vi "Read JSON from File.vi"(8 "error in (no error)":errorcluster, 11 "File Path":path) -> (0 "error out":errorcluster, 3 "<JSON>Config":string)   [LabVIEW 2023, in "HAL GOOP4.lvlib" / "Measure and Stimulus Subsystems.lvclass"]
uses:
  Measure and Stimulus Subsystems.lvclass
  <vilib>/Utility/error.llb/Error Cluster From Error Code.vi
  <vilib>/ErrorRing/Error Ring.xnode
  Measure and Stimulus Subsystems.lvclass/Measure and Stimulus Subsystems.ctl
  <vilib>/JDP Science/JSONtext/Config Files/Config File.lvclass
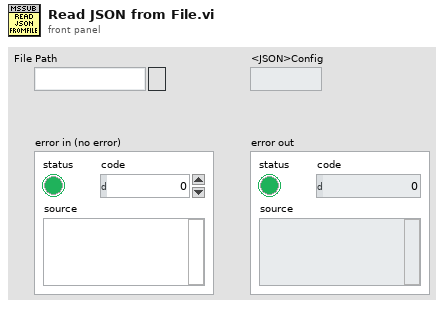
[diagram p1: front panel]
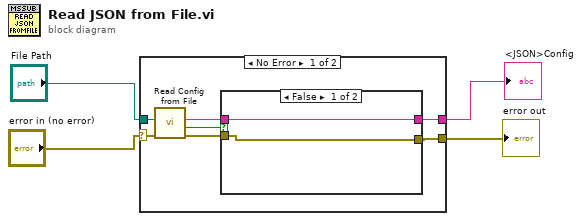
[diagram p0: block diagram]
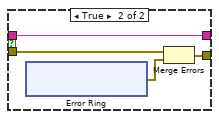
[diagram p2: hidden frame]
diagram:
  n1 = case shown="No Error" "error in (no error)" {
    selector: "error in (no error)" -> [w5 w23]
    tunnel: [w11 w23] -> w4
    tunnel: [w10 _] -> w3
    tunnel: "File Path" -> [w6 _]
    frame No Error {
      n2 = call <vilib>:"Read Config from File.vi"("error in (no error)"=w5, "config file path"=w6) -> ("error out"=w8:errorcluster, "Template Used (file missing or corrupted)"=w7:bool, "<JSON>Config"=w9:string)  [unwired: 6 in, 1 out]
      n3 = case shown="False" w7 {
        tunnel: w8 -> [w13 w17]
        tunnel: [w13 w15] -> w11
        tunnel: w9 -> [w12 w14]
        tunnel: [w12 w14] -> w10
        frame False {
        }
        frame True {
          n4 = xnode "Error Ring"() -> ("error out"=w16:errorcluster)
          n5 = Merge Errors(w17, w16) -> (w15:errorcluster)
        }
      }
    }
    frame Error {
    }
  }
  "error out" <- w4
  "<JSON>Config" <- w3
